vi "GetSystemTimeZone.vi"(11 "Error in":errorcluster caption="Error in (no error)") -> (4 "System Timezone Name":string, 6 "System Timezone Descriptor":string, 8 "UTC Offset":dbl, 15 "Error out":errorcluster)   [LabVIEW 2017, in "GPTiming.lvlib"]
doc: "Queries the (Windows only) system for currently set <B>System Timezone Name</B>.\n\nThis VI runs only if there is no error on <B>Error in</B>.\n\nSteen Schmidt\nGPower\n4/2 2017"
uses:
  GPTiming.lvlib
  Error/GPError.lvlib
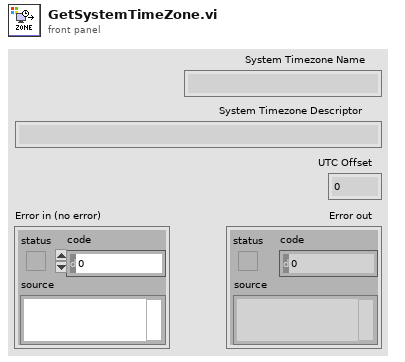
[diagram p1: front panel]
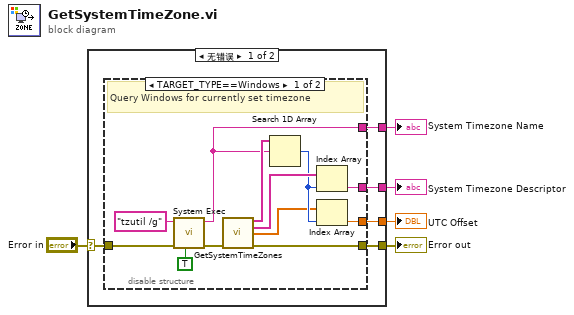
[diagram p0: block diagram]
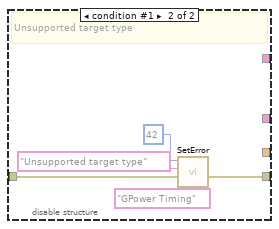
[diagram p2: hidden frame]
diagram:
  n1 = case shown="无错误" "Error in" {
    selector: "Error in" -> [w10 w28]
    tunnel: [w9 w28] -> w5
    tunnel: [w8 _] -> w4
    tunnel: [w7 _] -> w3
    tunnel: [w6 _] -> w2
    frame No Error {
      n2 = disable-structure shown="TARGET_TYPE==Windows" {
        disable-tunnel: w10 -> [w15 w25]
        disable-tunnel: [w14 w23] -> w9
        disable-tunnel: [w13 _] -> w8
        disable-tunnel: [w12 _] -> w7
        disable-tunnel: [w11 _] -> w6
        frame condition #0 (active) {
          # "Query Windows for currently set timezone"
          n3 = call <vilib>:"System Exec.vi"("run minimized? (F)"=TRUE, "error in (no error)"=w15, "command line"="tzutil /g") -> ("error out"=w18:errorcluster, "standard output"=w11:string)  [unwired: 5 in, 2 out]
          n4 = call "GetSystemTimeZones.vi"("Error in"=w18) -> ("System Timezone Names"=w19:string[], "System Timezone Descriptors"=w22:string[], "UTC Offsets"=w20:dbl[], "Error out"=w14:errorcluster)  [unwired: 11 in]
          n5 = Search 1D Array(1D array=w19, element=w11) -> (index of element=w21:i32)  [unwired: 1 in]
          n6 = Index Array(array=w22, index=w21) -> (element=w12:string)
          n7 = Index Array(array=w20, index=w21) -> (element=w13:dbl)
        }
        frame condition #1 {
          # "Unsupported target type"
          n8 = call "SetError.vi"("Error label"="GPower Timing", "Error in"=w25, "Error description"="Unsupported target type", "Error code"=42) -> ("Error out"=w23:errorcluster)  [unwired: 7 in]
        }
      }
    }
    frame Error {
    }
  }
  "Error out" <- w5
  "System Timezone Name" <- w2
  "UTC Offset" <- w4
  "System Timezone Descriptor" <- w3
